vi "Create_notification.vi"(11 "name":string="print") -> (3 "notification":i32)   [LabVIEW 2011]
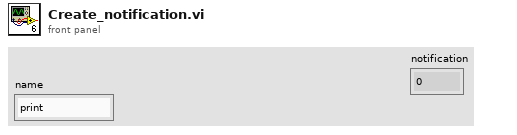
[diagram p1: front panel]
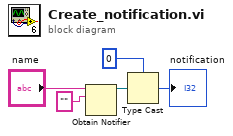
[diagram p0: block diagram]
diagram:
  n1 = Obtain Notifier(name (unnamed)="name", notification data type="" ("名称（未命名）")) -> (notifier out=w3:refnum<notifier>)  [unwired: 2 in, 2 out]
  n2 = Type Cast(type=0, x=w3) -> (*(type *) &x=→"notification":i32)
